vi "Setup Main.vi"(8 "error in (no error)":errorcluster, 9 "Path":path, 10 "Name":string) -> (0 "error out":errorcluster, 3 "Launcher out":refnum<class "Launcher.lvclass">)   [LabVIEW 2023, in "Launcher.lvlib" / "Launcher.lvclass"]
uses:
  Library/Launcher.lvclass
  Library/Launcher.lvclass/Launcher.ctl
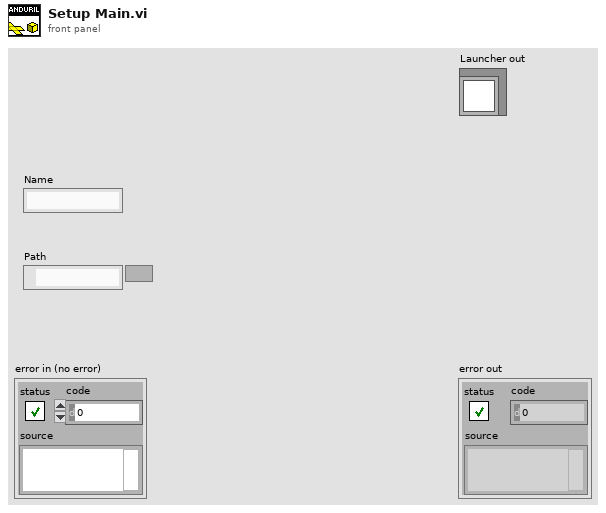
[diagram p1: front panel]
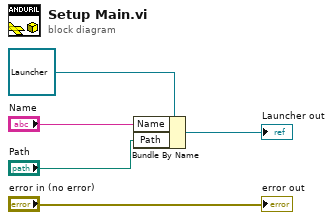
[diagram p0: block diagram]
diagram:
  n1 = Bundle By Name(cluster=refnum<class "Launcher.lvclass"> refnum ("Launcher in"), "Name"="Name", "Path"="Path") -> (→"Launcher out":refnum<class "Launcher.lvclass">)
  "error out" <- "error in (no error)"
